vi "Copy Template to Express VI.vi"(8 "error in (no error)":errorcluster, 11 "Refs in":T1) -> (0 "error out":errorcluster, 3 "Refs":T1)   [LabVIEW 2020, in "FlexBlocks.lvlib"]
uses:
  FlexBlocks.lvlib
  Scripting Refs.ctl
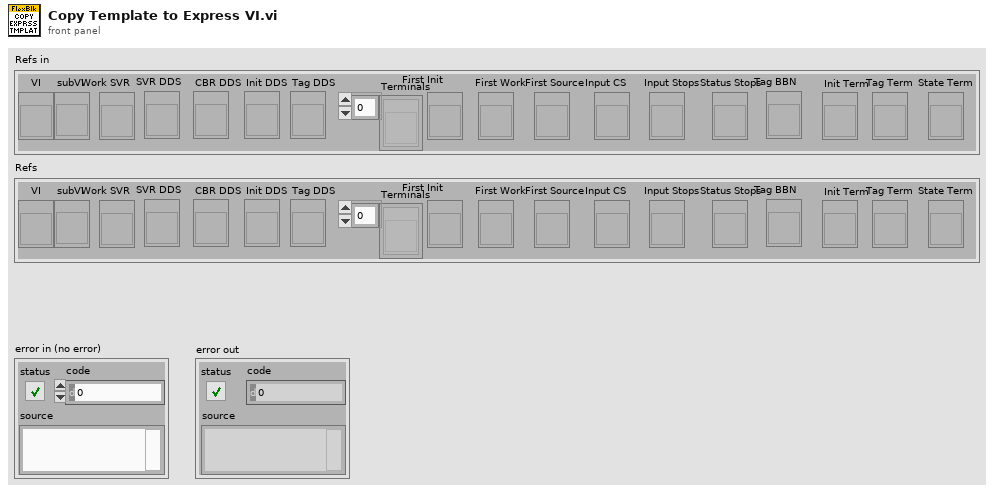
[diagram p1: front panel]
types:
  T1 = typedef "FlexBlocks.lvlib/Scripting Refs.ctl" = cluster{"VI":refnum<vi>, "subVI":refnum<vi>, "Work SVR":refnum<vi>, "SVR DDS":refnum<vi>, "CBR DDS":refnum<vi>, "Init DDS":refnum<vi>, "Tag DDS":refnum<vi>, "Terminals":refnum<vi>[], "First Init":refnum<vi>, "First Work":refnum<vi>, "First Source":refnum<vi>, "Input CS":refnum<vi>, "Input Stops":refnum<vi>, "Status Stops":refnum<vi>, "Tag BBN":refnum<vi>, "Init Term":refnum<vi>, "Tag Term":refnum<vi>, "State Term":refnum<vi>}
  T2 = typedef "FlexBlocks.lvlib/Paths.ctl" = cluster{"FlexBlocks":path, "Workers Root":path, "Specialized Editors":path, "Worker Template":path, "Editor Template":path, "Express Template":path, "Control Ref Vim":path}
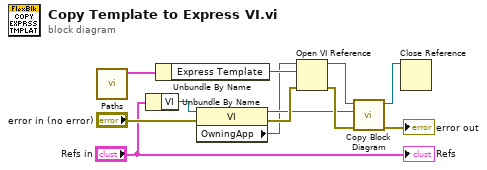
[diagram p0: block diagram]
diagram:
  n1 = call "Paths.vi"() -> ("Paths"=w10:T2)  [unwired: 11 in]
  n2 = Unbundle By Name("Refs in") -> ("VI"=w3:refnum<vi>)
  n3 = Unbundle By Name(w10) -> ("Express Template"=w9:path)
  n4 = property class="VI"(reference=w3, error in="error in (no error)") -> (reference out=w8:refnum<vi>, error out=w11:errorcluster, "OwningApp"=w4:refnum<vi>)
  n5 = Open VI Reference(application reference (local)=w4, vi path=w9, error in (no error)=w11) -> (vi reference=w7:refnum<vi>, error out=w12:errorcluster)  [unwired: 3 in]
  n6 = call "Copy Block Diagram.vi"("error in (no error)"=w12, "Dest In"=w8, "Source In"=w7) -> ("error out"=→"error out":errorcluster, "Source"=w6:refnum<vi>)  [unwired: 6 in, 1 out]
  n7 = Close Reference(reference=w6) -> ()  [unwired: 1 in, 1 out]
  "Refs" <- "Refs in"
